vi "Lidar_dis.vi"() -> ()   [LabVIEW 2014]
panel:
  out "双精度浮点数 2":dbl
  out "双精度浮点数":dbl
  out "布尔":bool
  out "Lidar_size":u8
  in  "distance":dbl[](array[numeric])
  in  "angle":dbl[](array[numeric])
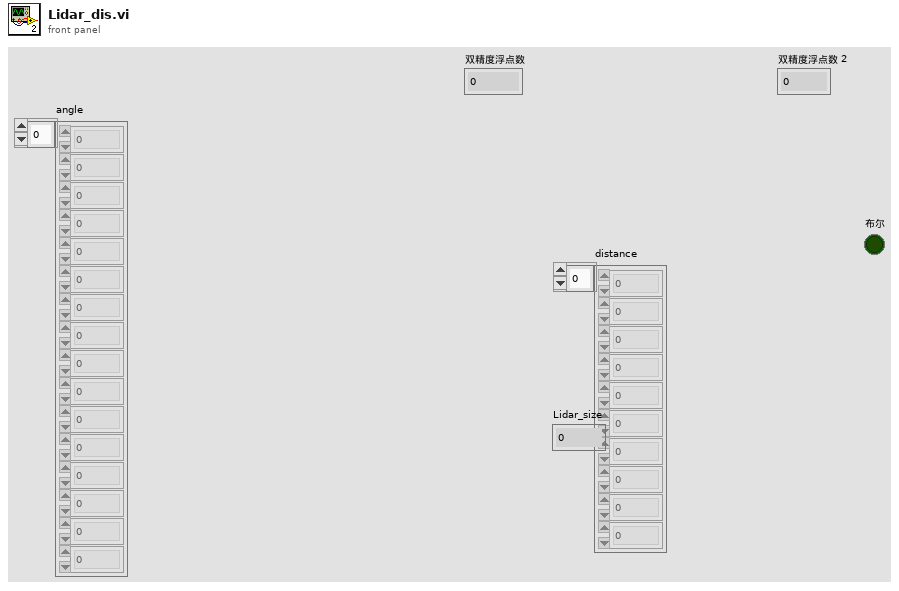
[diagram p1: front panel]
types:
  T1 = cluster{"quality":u8, "angle":u16, "distance\n":u16}
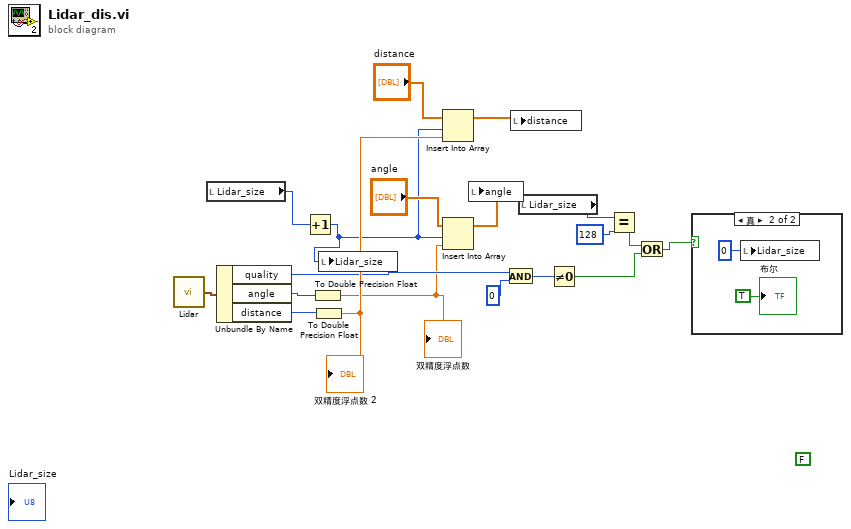
[diagram p0: block diagram]
diagram:
  (unwired) FALSE
  n1 = call "Lidar.vi"() -> ("输出簇"=w19:T1)  [unwired: 1 in]
  n2 = local read "Lidar_size"() -> (w5:u8)
  n3 = Unbundle By Name(w19) -> ("quality"=w7:u8, "angle"=w8:u16, "distance"=w10:u16)
  n4 = Increment(x=w5) -> (x+1=w3:u8)
  n5 = To Double Precision Float(number=w8) -> (double precision float=w4:dbl)
  "双精度浮点数" <- w4
  n6 = To Double Precision Float(number=w10) -> (double precision float=w9:dbl)
  "双精度浮点数 2" <- w9
  n7 = local write "Lidar_size"(w3) -> ()
  n8 = Insert Into Array(array="distance", index=w3, new element=w9) -> (w1:dbl[])
  n9 = Insert Into Array(array="angle", index=w3, new element=w4) -> (w2:dbl[])
  n10 = local write "angle"(w2) -> ()
  n11 = And(x=w7, y=u8 0) -> (x .and. y?=w14:u8)
  n12 = local write "distance"(w1) -> ()
  n13 = local read "Lidar_size"() -> (w16:u8)
  n14 = Not Equal To 0?(x=w14) -> (x != 0?=w12:bool)
  n15 = Equal?(x=w16, y=u8 128) -> (x = y?=w13:bool)
  n16 = Or(x=w13, y=w12) -> (x .or. y?=w11:bool)
  n17 = case shown="真" w11 {
    frame False {
    }
    frame True {
      n18 = local write "Lidar_size"(u8 0 ("Lidar_size")) -> ()
      "布尔" <- TRUE ("布尔")
    }
  }
